vi "DHE_SetROI.vi"(0 "refnum":i32=2048, 1 "xsize":u16, 2 "ysize":u16, 7 "xstart":u16, 9 "ystart":u16, 11 "error in (no error)":errorcluster, 12 "new roi":bool, 13 "full roi":bool) -> (4 "fd out":i32, 6 "return value":i32, 8 "X total size":u16, 10 "Y total size":u16, 14 "DET_READ_TIME":sgl=3.5 format="%.2f", 15 "error out":errorcluster)   [LabVIEW 2016]
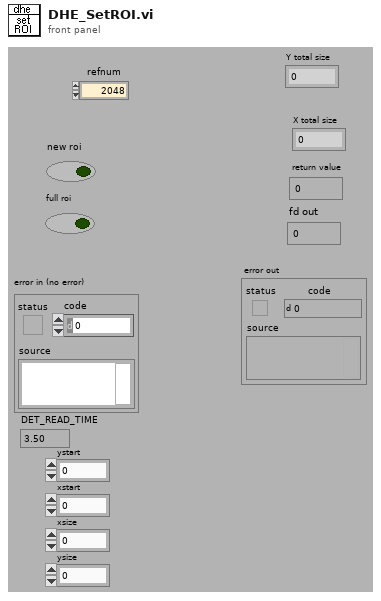
[diagram p1: front panel]
types:
  T1 = typedef "GEOM_CorrectedFPA.ctl" = cluster{"readmode":string, "amplifiers":cluster{"number":i32, "xstart":i32, "ystart":i32}[], "totxsize":i32, "totysize":i32, "maxxdim":i32, "maxydim":i32, "numxamps":i32, "numyamps":i32, "totxdata":i32, "totydata":i32, "xdataamp":i32, "ydataamp":i32, "totpixels":i32}
  T2 = typedef "GEOM_Amplifier.ctl" = cluster{"number":i32, "type":T3, "rotated":i16, "fliped":u16, "FPAcoord":cluster{"xstart":i32, "ystart":i32}, "Physical_size":cluster{"columns":i32, "rows":i32}, "predata":cluster{"columns":i32, "rows":i32}, "postdata":cluster{"columns":i32, "rows":i32}, "Req ROIs":T4, "Corr ROI":T4, "Detnumber":i32, "ampID":string, "discard":i32}
  T3 = typedef "GEOM_AmpType.ctl" = u16
  T4 = typedef "GEOM_ROI.ctl" = T5[]
  T5 = typedef "GEOM_Coords.ctl" = cluster{"xstart":u32, "ystart":u32, "xsize":u32, "ysize":u32}
  T6 = typedef "DatabaseHand_RefNum.ctl" = refnum<vi>
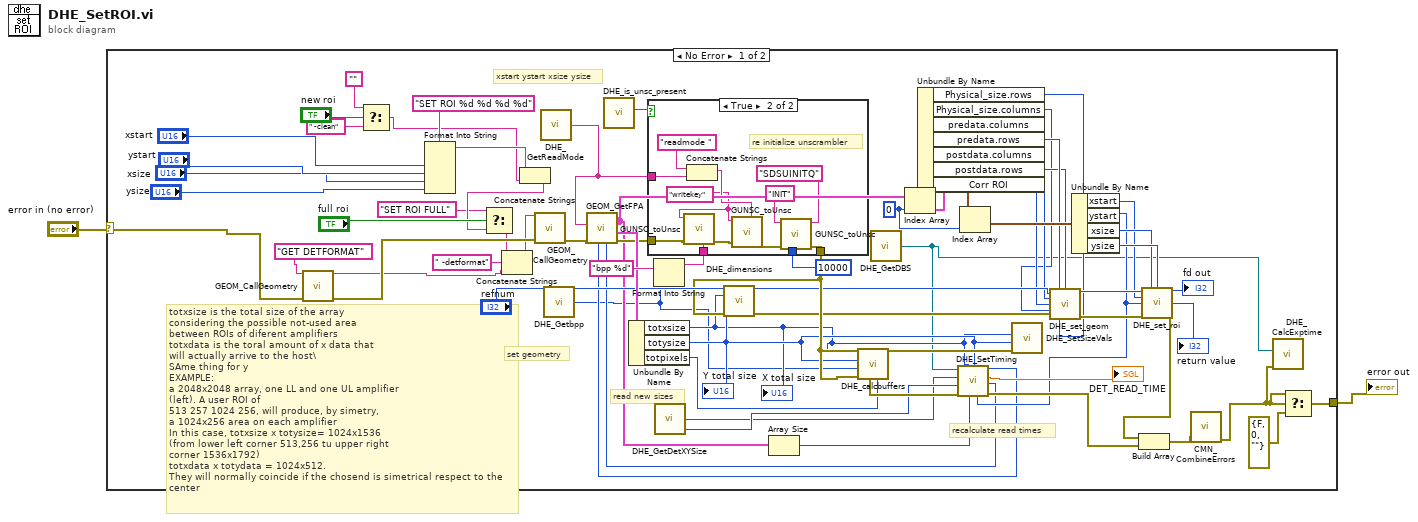
[diagram p0: block diagram]
diagram:
  n1 = case shown="No Error" "error in (no error)" {
    selector: "error in (no error)" -> [w10 w85]
    tunnel: [w24 w85] -> w1
    frame No Error {
      w47 = 0 ("index")
      # "totxsize is the total size of the array\nconsidering the possible not-used area\nbetween ROIs of diferent amplifiers\ntotxdata is the toral amount of x data that\nwill actually arrive to the host\\\nSAme thing for y\nEXAMPLE:\na 2048x2048 array, one LL and one UL amplifier\n(left). A user ROI of\n513 257 1024 256, will produce, by simetry, \na 1024x256 area on each amplifier\nIn this case, totxsize x totysize= 1024x1536\n(from lower left corner 513,256 tu upper right\ncorner 1536x1792)\ntotxdata x totydata = 1024x512.\nThey will normally coincide if the chosend is simetrical respect to the center"
      # "xstart ystart xsize ysize"
      # "recalculate read times"
      # "read new sizes"
      # "set geometry"
      n2 = call "GEOM_CallGeometry.vi"("Command"="GET DETFORMAT", "error in (no error)"=w10) -> ("ImmedReplyString"=w5:string, "error out"=w9:errorcluster)  [unwired: 12 out]
      n3 = Select(t="", s="new roi", f=" -clean") -> (s? t:f=w50:string)
      n4 = Format Into String(format string="SET ROI %d %d %d %d", "xstart", "ystart", "xsize", "ysize") -> (resulting string=w53:string)  [unwired: 2 in, 1 out]
      n5 = Concatenate Strings(w53, w50) -> (w15:string)
      n6 = Select(t="SET ROI FULL", s="full roi", f=w15) -> (s? t:f=w8:string)
      n7 = Concatenate Strings(w8, " -detformat" ("string"), w5) -> (w7:string)
      n8 = call "GEOM_CallGeometry.vi"("Command"=w7, "error in (no error)"=w9) -> ("error out"=w66:errorcluster)  [unwired: 13 out]
      n9 = call "DHE_GetReadMode.vi"() -> ("DHE_ReadMode"=w20:string)  [unwired: 9 out]
      n10 = call "DHE_Getbpp.vi"() -> ("DHE_bpp"=w19:i32)  [unwired: 9 out]
      n11 = call "GEOM_GetFPA.vi"("error in (no error)"=w66, "readmode"=w20) -> ("error out"=w64:errorcluster, "CorrectedFPACoord"=w65:T1, "amplifiers"=w38:T2[], "numyamps"=w21:i32, "numxamps"=w22:i32)  [unwired: 1 in, 4 out]
      n12 = call "DHE_is_unsc_present.vi"() -> ("value"=w13:bool)  [unwired: 1 in, 10 out]
      n13 = Unbundle By Name(w65) -> ("totxsize"=w31:i32, "totysize"=w32:i32, "totpixels"=w12:i32)
      "Y total size" <- w32
      "X total size" <- w31
      n14 = Format Into String(format string="bpp %d", w19) -> (resulting string=w63:string)  [unwired: 2 in, 1 out]
      n15 = case shown="True" w13 {
        tunnel: 10000 ("ms timeout (-1)") -> [_ w79]
        tunnel: w64 -> [w72 w78]
        tunnel: w63 -> [_ w75]
        tunnel: [w72 w74] -> w60
        tunnel: w20 -> [_ w73]
        frame False {
        }
        frame True {
          w76 = "writekey" ("command")
          # "re initialize unscrambler"
          n16 = call "GUNSC_toUnsc.vi"("key"=w75, "error in (no error)"=w78, "command"=w76) -> ("error out"=w77:errorcluster)  [unwired: 6 in, 2 out]
          n17 = Concatenate Strings("readmode " ("string"), w73) -> (w82:string)
          n18 = call "GUNSC_toUnsc.vi"("key"=w82, "error in (no error)"=w77, "command"=w76) -> ("error out"=w84:errorcluster)  [unwired: 6 in, 2 out]
          n19 = call "GUNSC_toUnsc.vi"("responseQ"="SDSUINITQ", "bpp"=w79, "error in (no error)"=w84, "command"="INIT") -> ("error out"=w74:errorcluster)  [unwired: 5 in, 2 out]
        }
      }
      n20 = call "DHE_GetDetXYSize.vi"() -> ("DHE_DetYsize"=w17:i32, "DHE_DetXsize"=w18:i32)  [unwired: 8 out]
      n21 = call "DHE_dimensions.vi"("fd"="refnum", "Columns"=w31, "Rows"=w32, "error in (no error)"=w60) -> ("fd out"=w57:i32, "error out"=w33:errorcluster)  [unwired: 10 out]
      n22 = Array Size(array=w38) -> (size(s)=w62:i32)
      n23 = call "DHE_calcbuffers.vi"("totpixelsin"=w12, "error in (no error)"=w60, "bpp"=w19, "nrows"=w32, "ncols"=w31) -> ("error out"=w68:errorcluster)  [unwired: 1 in, 5 out]
      n24 = call "DHE_GetDBS.vi"() -> ("DHE_DBSRef"=w3:T6)  [unwired: 9 out]
      n25 = Index Array(array=w38, index=w47) -> (element=w46:T2)
      n26 = Unbundle By Name(w46) -> ("Physical_size.rows"=w29:i32, "Physical_size.columns"=w30:i32, "predata.columns"=w35:i32, "predata.rows"=w37:i32, "postdata.columns"=w34:i32, "postdata.rows"=w36:i32, "Corr ROI"=w45:T4)
      n27 = Index Array(array=w45, index=w47) -> (element=w44:T5)
      n28 = call "DHE_SetSizeVals.vi"("error in"=w60, "ytotsize"=w32, "xtotsize"=w31) -> ()  [unwired: 9 out]
      n29 = call "DHE_set_geom.vi"("fd"=w57, "ypredata"=w37, "ypostdata"=w36, "xpredata"=w35, "xpostdata"=w34, "xdata"=w30, "error in (no error)"=w33, "ydata"=w29) -> ("fd out"=w56:i32, "error out"=w55:errorcluster)  [unwired: 6 out]
      n30 = Unbundle By Name(w44) -> ("xstart"=w41:u32, "ystart"=w23:u32, "xsize"=w42:u32, "ysize"=w43:u32)
      n31 = call "DHE_SetTiming.vi"("num of Y amps"=w21, "num of X amps"=w22, "yroi start"=w23, "roi rows"=w32, "Num of amps"=w62, "roi cols"=w31, "error in"=w68, "totysize"=w18, "totxsize"=w17, "Database RefNum out"=w3) -> ("errorout"=w26:errorcluster, "DET_READ_TIME"=→"DET_READ_TIME":sgl)
      n32 = call "DHE_set_roi.vi"("fd"=w56, "xlenght"=w42, "ylenght"=w43, "xstart"=w41, "ystart"=w23, "error in (no error)"=w55) -> ("fd out"=→"fd out":i32, "return value"=→"return value":i32, "error out"=w28:errorcluster)  [unwired: 7 out]
      n33 = Build Array(w28, w26) -> (w27:errorcluster[])
      n34 = call "CMN_CombineErrors.vi"("Errors"=w27) -> ("error out"=w4:errorcluster)  [unwired: 10 out]
      n35 = call "DHE_CalcExptime.vi"("error in (no error)"=w4, "DHE_DBSRef"=w3) -> ()  [unwired: 10 out]
      n36 = Select(t=w4, s=w4, f=errorcluster {"status"=FALSE, "code"=0, "source"=""}) -> (s? t:f=w24:errorcluster)
    }
    frame Error {
    }
  }
  "error out" <- w1
